vi "Motion Profile Global Variable.vi"() -> ()   [LabVIEW 2017]
panel:
  in  "CSV File Name":string
  out "Reset Motion Profile Points":bool
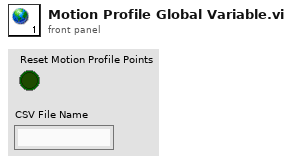
[diagram p1: front panel]
diagram:
